vi "位置转换.vi"(8 "error in (no error)":errorcluster, 11 "In":dbl) -> (0 "error out":errorcluster, 3 "Out":dbl)   [LabVIEW 2020, in "输出轴伺服.lvlib"]
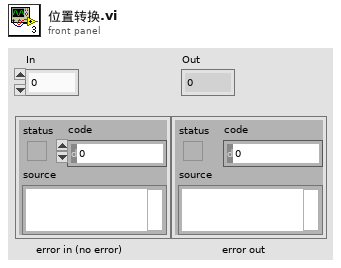
[diagram p1: front panel]
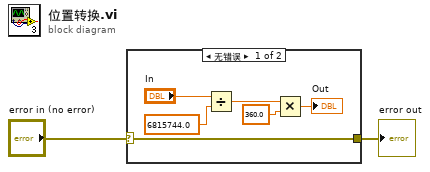
[diagram p0: block diagram]
diagram:
  n1 = case shown="无错误" "error in (no error)" {
    selector: "error in (no error)" -> [w3 w9]
    tunnel: [w3 w9] -> w1
    frame No Error {
      n2 = Divide(x="In", y=6815744.0) -> (x/y=w7:dbl)
      n3 = Multiply(x=w7, y=360.0) -> (x*y=→"Out":dbl)
    }
    frame Error {
    }
  }
  "error out" <- w1
